vi "EnFlo_Turntable_Control.vi"(3 "Mode":T5, 5 "Traverse line In":T2={"Start X"=0.0, "Start Y"=nan, "Start Z"=nan, "End X"=nan, "End Y"=nan, "End Z"=nan, "nPoints"=0, "Spacing"=enum."N/A", "Filename"=path "  ---------", "Tunnel Speed"=nan, "Averaging time (mins)"=nan, "Extra Commands"="!Datum Image = Datum_Turntable.xls", "Carrier_1 Q (l/min)"=nan, "Carrier_2 Q (l/min)"=nan, "Trace Gas Concentration (%)"=nan, "Specific Arguments"="EnFlo_Turntable_Control.vi", "Comments"="", "Row No"=0, "Row Type Selector"=enum."Run VI Named:", "EstCompl"="09:40  12-04-2016", "Row Duration (mins)"=0.6666666666666666, "nValidPoints"=0, "Meas Setup File"="Trav_Cam_Picture.xls"} {"Carrier_2 Q (l/min)" format="%#.2f"; "Row Duration (mins)" format="%#.1f"; "Row No" min=0; "Trace Gas Concentration (%)" min=0.0 format="%#_4f"; "Carrier_1 Q (l/min)" format="%#.4f"; "Start X" format="%#.2f"; "Start Y" format="%#.2f"; "Start Z" format="%#.2f"; "End X" format="%#.2f"; "End Y" format="%#.2f"; "End Z" format="%#.2f"; "Tunnel Speed" format="%#.2f"; "Averaging time (mins)" min=0.0 format="%#.2f"}) -> (0 "Error Message":string, 1 "Status":T1, 2 "Traverse line Out":T2={"Start X"=0.0, "Start Y"=nan, "Start Z"=nan, "End X"=nan, "End Y"=nan, "End Z"=nan, "nPoints"=0, "Spacing"=enum."N/A", "Filename"=path "  ---------", "Tunnel Speed"=nan, "Averaging time (mins)"=nan, "Extra Commands"="!Datum Image = Datum_Turntable.xls", "Carrier_1 Q (l/min)"=nan, "Carrier_2 Q (l/min)"=nan, "Trace Gas Concentration (%)"=nan, "Specific Arguments"="EnFlo_Turntable_Control.vi", "Comments"="", "Row No"=0, "Row Type Selector"=enum."Run VI Named:", "EstCompl"="09:40  12-04-2016", "Row Duration (mins)"=0.6666666666666666, "nValidPoints"=0, "Meas Setup File"="Trav_Cam_Picture.xls"} {"Carrier_2 Q (l/min)" format="%#.2f"; "Row Duration (mins)" format="%#.1f"; "Row No" min=0; "Trace Gas Concentration (%)" min=0.0 format="%#_4f"; "Carrier_1 Q (l/min)" format="%#.4f"; "Start X" format="%#.2f"; "Start Y" format="%#.2f"; "Start Z" format="%#.2f"; "End X" format="%#.2f"; "End Y" format="%#.2f"; "End Z" format="%#.2f"; "Tunnel Speed" format="%#.2f"; "Averaging time (mins)" min=0.0 format="%#.2f"})   [LabVIEW 2022 SP3]
uses:
  Gen Trav/Traverse_cluster.ctl
  Gen Trav/Spacing.ctl
  Controls/Multi_run_mode.ctl
  Controls/User_Specific_mode.ctl
  Gen Trav/Multi_Run_Status.ctl
  Gen Trav/Trav_mode.ctl
  Controls/Tunnel_Coordinates.ctl
  ADAM Client/Sub VIs/ADAM Controls/Quick_local_ADAM_Table.ctl
  Controls/Setup.ctl
  Controls/Save_Data.ctl
  Camera Server/Camera enum/Camera resolution.ctl
  ADAM Client/Sub VIs/ADAM Controls/Update_scan_value.ctl
  Globals/Trav_pos_global.vi
  Globals/Extra_Commands_Global.vi
  Globals/Constants_global.vi
  Globals/Dynamic_call_global.ph.vi
panel:
  out "File Traverse Parking info comes from":path
  out "Traverse Parking Positions":string[][](table)
  out "Datum Filename":string
  out "Turntable image angle error":bool
  in  "max num of moves":i32=10
  out "Ratio of Error to move":sgl=0.8
  in  "stop":bool
  out "Turntable Angle":sgl format="%0.2f"
  out "Error in Turntable":sgl(graph)
  out "Angle Tolerance":sgl=0.02 format="%#_13g"
  out "Turntable Error":sgl
  out "Motor Position (Angle)":sgl(graph)
  out "Demanded Deg":sgl format="%#.4f"
  out "Correct Position":bool=TRUE
  out "Drive needs relaxing?":bool
  out "Relax Drive":sgl=0.25
  out "+ve Rotation":bool
  out "Motor Current Position":sgl
  # "X           Y          Z"
  # "Start"
  # "End"
  # "X           Y          Z"
  # "Start"
  # "End"
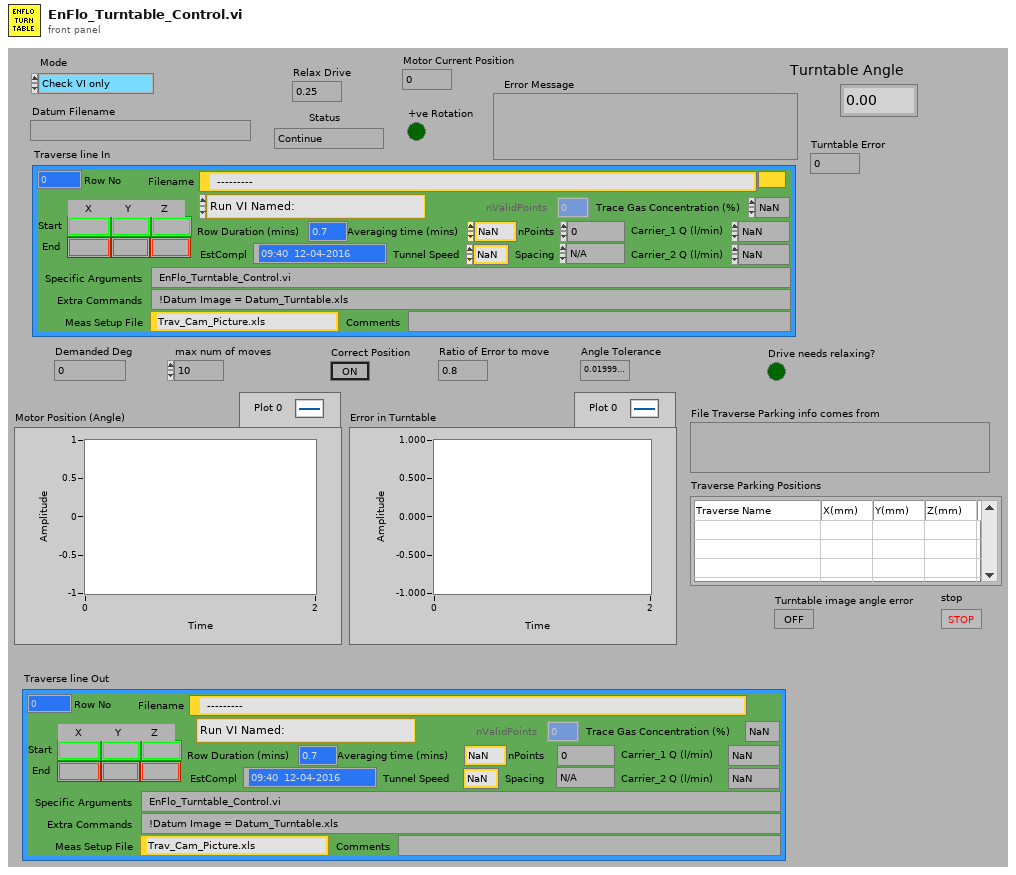
[diagram p1: front panel]
types:
  T1 = typedef "Multi_Run_Status.ctl" = enum16{"Continue", "Continue with Error", "Jump to Next Point", "Jump to Next Row", "Jump To Fall Back", "Terminate Run"}
  T2 = typedef "Traverse_cluster.ctl" = cluster{"Start X":sgl, "Start Y":sgl, "Start Z":sgl, "End X":sgl, "End Y":sgl, "End Z":sgl, "nPoints":i32, "Spacing":T3, "Filename":path, "Tunnel Speed":dbl, "Averaging time (mins)":dbl, "Extra Commands":string, "Carrier_1 Q (l/min)":dbl, "Carrier_2 Q (l/min)":dbl, "Trace Gas Concentration (%)":dbl, "Specific Arguments":string, "Comments":string, "Row No":i32, "Row Type Selector":T4, "EstCompl":string, "Row Duration (mins)":dbl, "nValidPoints":i32, "Meas Setup File":string}
  T3 = typedef "Spacing.ctl" = enum16{"Linear", "Log", "Gauss", "Specified", "N/A"}
  T4 = typedef "Multi_run_mode.ctl" = enum16{"Move Traverse Only", "Set Tunnel Speed Only", "Set Source Only", "Set Measurement Conditions", "Single Measurement", "Vertical Profile", "Lateral Profile", "Longitudinal Profile", "Multi-Axis Profile", "Explore Volume", "Auto Calibrate", "Meas Fast FID Bkgnd", "Check Beam Power", "Scanning Valve Measurement", "Run VI Named:", "Set ADAM Ch", "Wait (minutes)", "Send Message", "Synchronize With:", "Fall Back to this Row", "Turn Off Row Repeating", "Traverse 3D Volume", "Blank Row", "Jump to Fall Back Row"}
  T5 = typedef "User_Specific_mode.ctl" = enum16{"Check VI only", "Run VI"}
  T6 = typedef "Trav_mode.ctl" = enum16{"Move traverse", "Read traverse position", "Teach Position"}
  T7 = typedef "Tunnel_Coordinates.ctl" = enum16{"Work in Tunnel Coordinates", "Work in Model Coordinates"}
  T8 = typedef "Quick_local_ADAM_Table.ctl" = enum16{"Read Global", "Load Global From ADAM Table", "Write Global"}
  T9 = typedef "Save_Data.ctl" = enum16{"Save No Data", "Save Data"}
  T10 = typedef "Setup.ctl" = enum16{"Run Program", "Show Setup", "Save Current Setup", "Setup Front Panel"}
  T11 = typedef "Update_scan_value.ctl" = cluster{"Channel Name":string, "New Value":dbl, "!Auto_Off":bool}
  T12 = typedef "Camera resolution.ctl" = u8
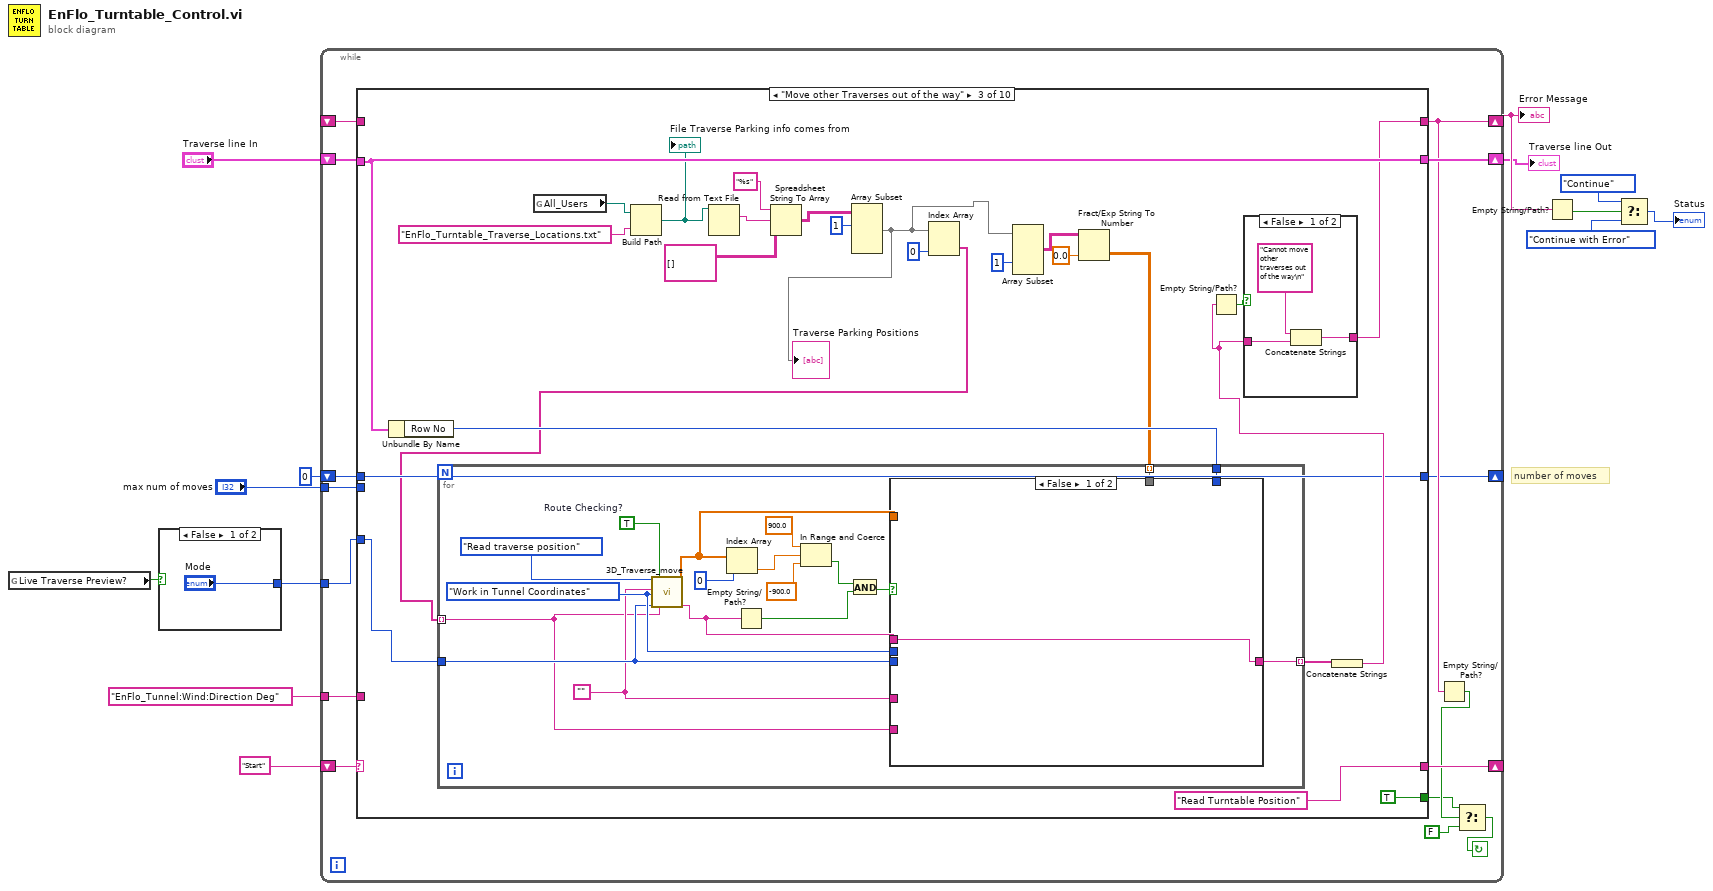
[diagram p0: block diagram]
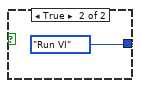
[diagram p2: hidden frame]
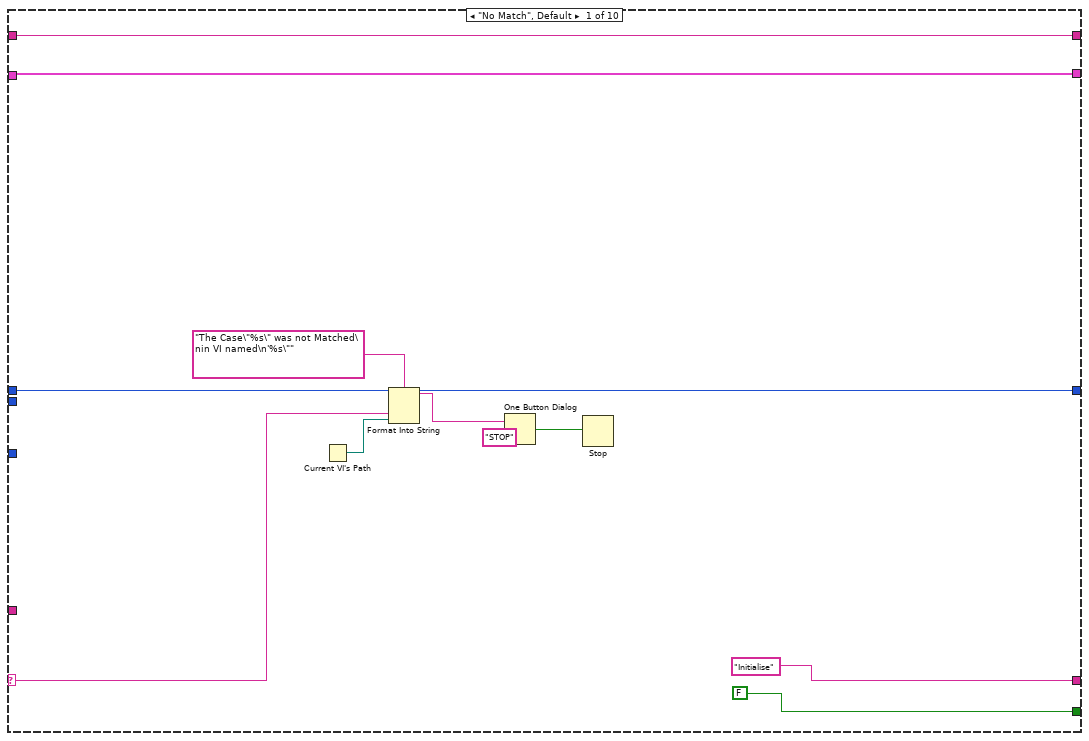
[diagram p3: hidden frame]
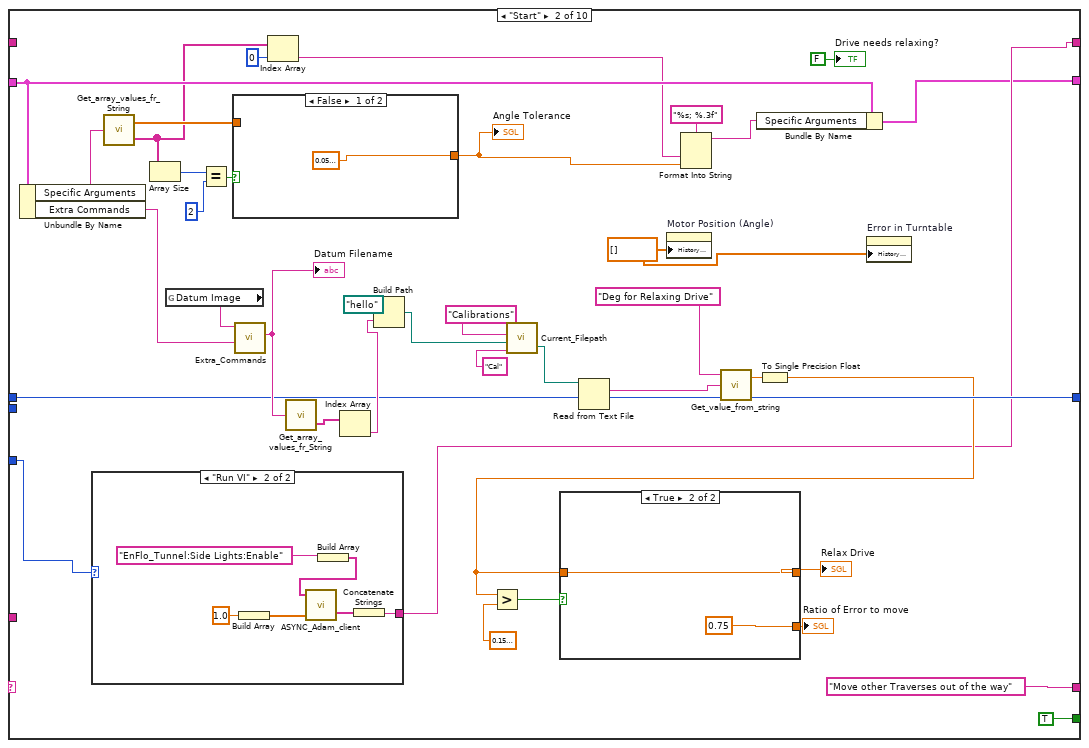
[diagram p4: hidden frame]
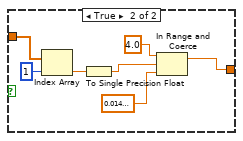
[diagram p5: hidden frame]
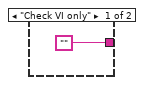
[diagram p6: hidden frame]
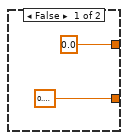
[diagram p7: hidden frame]
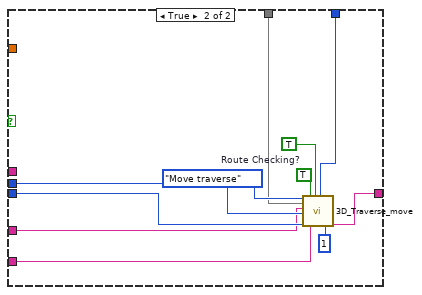
[diagram p9: hidden frame]
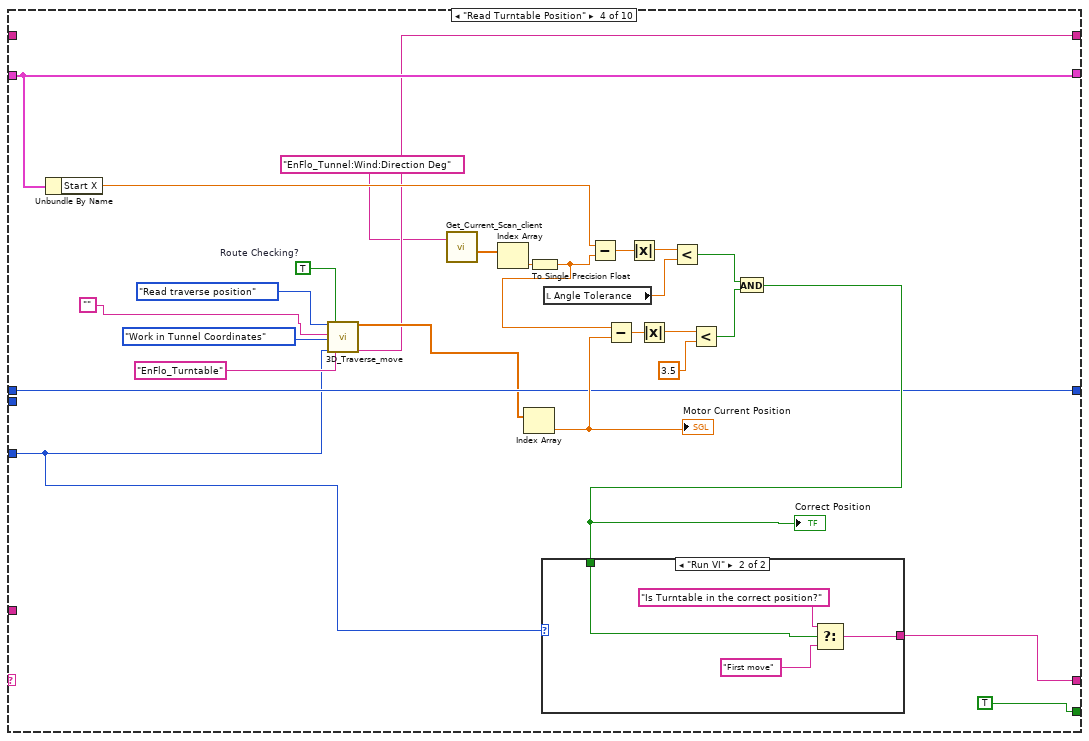
[diagram p10: hidden frame]
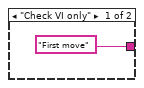
[diagram p11: hidden frame]
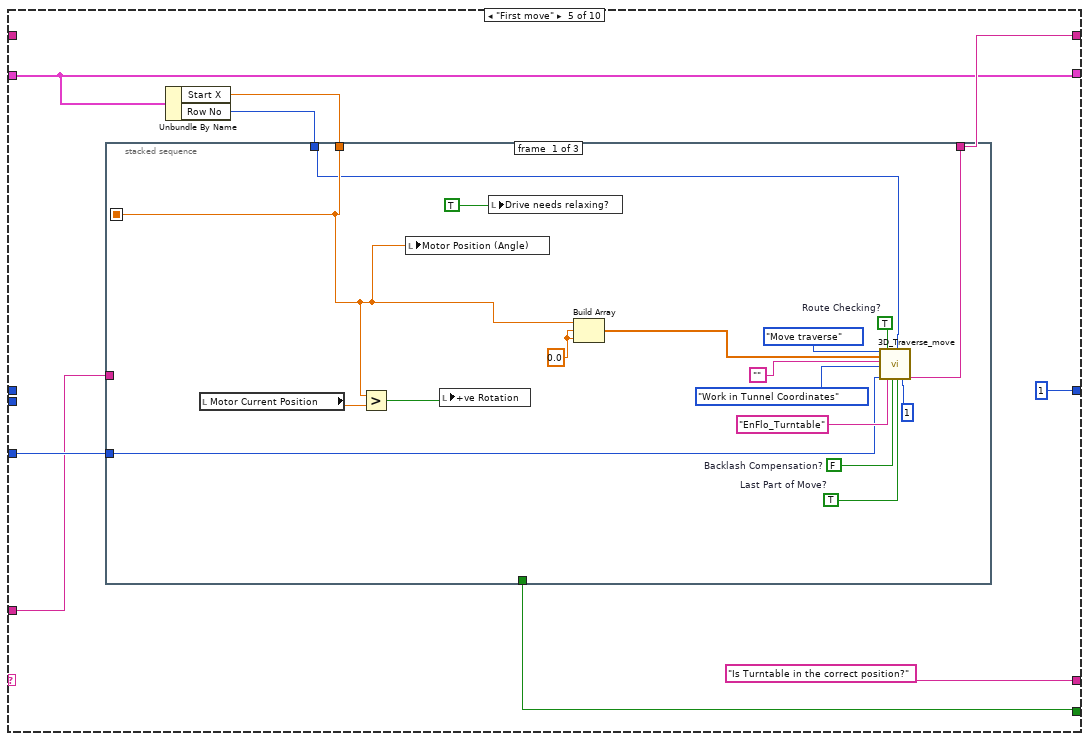
[diagram p12: hidden frame]
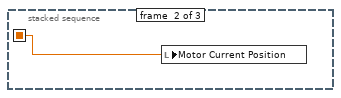
[diagram p13: hidden frame]
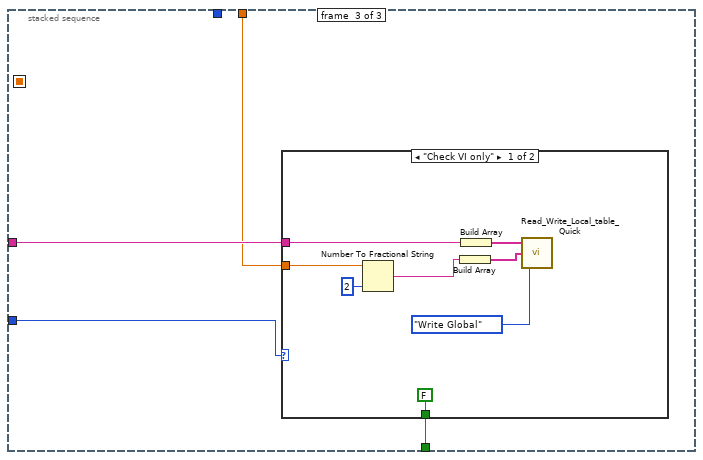
[diagram p14: hidden frame]
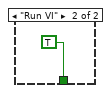
[diagram p15: hidden frame]
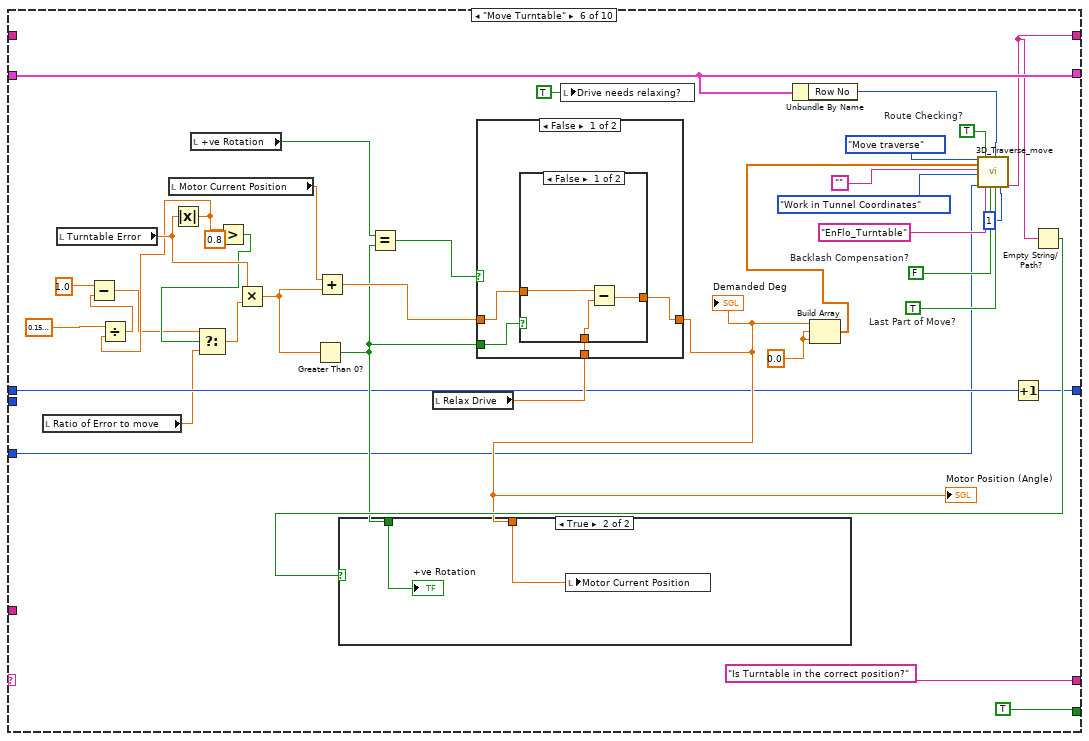
[diagram p16: hidden frame]
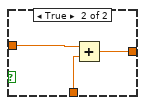
[diagram p17: hidden frame]
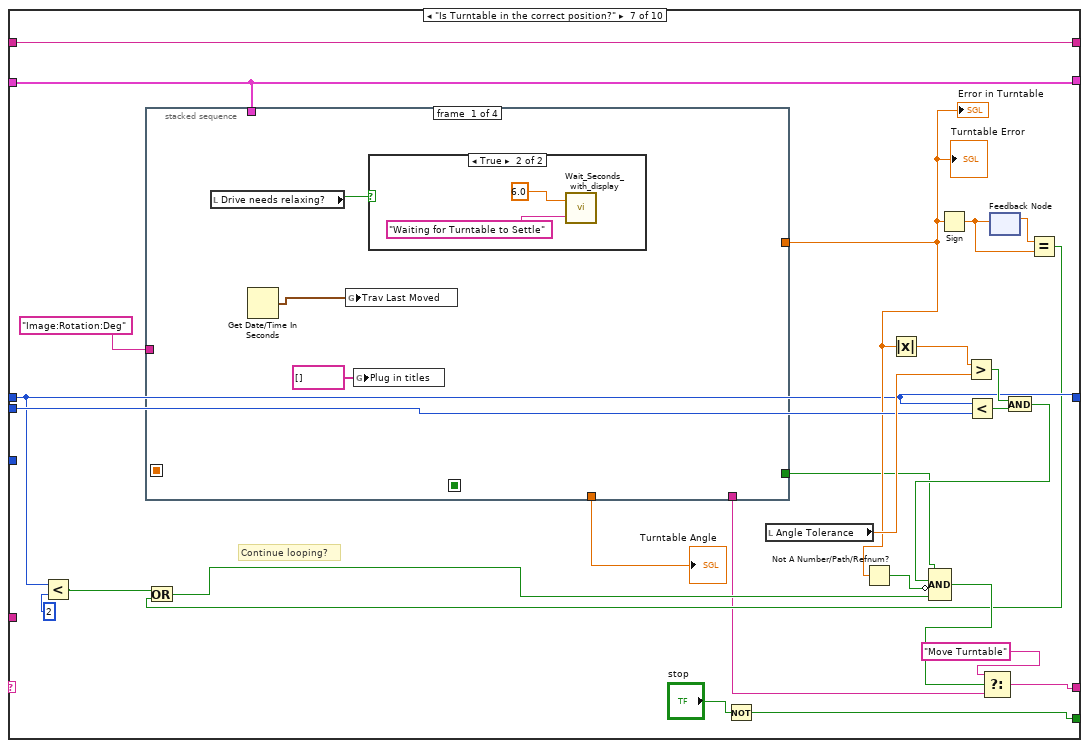
[diagram p20: hidden frame]
diagram:
  # "number of moves"
  n1 = global read "Trav_pos_global.vi" "Live Traverse Preview?"() -> (w4:bool)
  n2 = case shown="False" w4 {
    tunnel: ["Mode" User_Specific_mode."Run VI" ("Simulate/Run")] -> w3
    frame False {
    }
    frame True {
    }
  }
  n3 = while {
    shift-left: "Start" -> [w29]
    shift-right: [w30] -> _
    shift-right: [w27] -> w1
    shift-left: "Traverse line In" -> [w28]
    shift-right: [w25] -> w12
    shift-left: _ -> [w26]
    shift-right: [w20] -> _
    shift-left: 0 -> [w19]
    tunnel: "max num of moves" -> [w18]
    tunnel: w3 -> [w17]
    tunnel: "EnFlo_Tunnel:Wind:Direction Deg" -> [w16]
    stop <- w22 continue-if-true
    n4 = case shown="\"Move other Traverses out of the way\"" w29 {
      selector: w29 -> [w32 _ _ _ _ _ _ _ _ _]
      tunnel: [FALSE TRUE TRUE TRUE w192 TRUE w302 TRUE TRUE FALSE] -> w23
      tunnel: ["Initialise" "Move other Traverses out of the way" "Read Turntable Position" ("f") w182 "Is Turntable in the correct position?" "Is Turntable in the correct position?" w305 "Relax Turntable Drive" "Update Adam Table" "End"] -> w30
      tunnel: w17 -> [_ w57 w123 w159 w197 w230 _ w357 w383 _]
      tunnel: w28 -> [w34 w49 w118 w184 w195 w265 w301 w376 w399 w424]
      tunnel: [w34 w42 w118 w184 w195 w265 w301 w376 w399 w424] -> w27
      tunnel: [w33 w55 w115 w162 w196 w233 w288 w359 w386 w418] -> w25
      tunnel: w26 -> [w33 _ _ _ _ _ w288 _ _ w419]
      tunnel: [w31 w58 w114 w168 1 w253 w287 1 w397 w420] -> w20
      tunnel: w19 -> [w31 w58 w114 w168 _ w252 w287 _ w397 w420]
      tunnel: w18 -> [_ _ _ _ _ _ w299 _ _ _]
      tunnel: w16 -> [_ _ _ _ w190 _ _ _ _ w415]
      frame "No Match", Default {
        n5 = Current VI's Path() -> (path=w36:path)
        n6 = Format Into String(format string="The Case\"%s\" was not Matched\nin VI named\n'%s\"" ("Format String"), w32, w36) -> (resulting string=w39:string)  [unwired: 2 in, 1 out]
        n7 = One Button Dialog(message=w39, button name ("OK")="STOP") -> (true=w37:bool)
        n8 = Stop(stop? (T)=w37) -> ()
      }
      frame "Start" {
        w78 = dbl[] [] ("History Data")
        n9 = Unbundle By Name(w49) -> ("Specific Arguments"=w54:string, "Extra Commands"=w77:string)
        n10 = case shown="\"Run VI\"" w57 {
          tunnel: ["" w89] -> w55
          frame "Check VI only" {
          }
          frame "Run VI" {
            n11 = Build Array(1.0 ("element")) -> (w94:dbl[])
            n12 = Build Array("EnFlo_Tunnel:Side Lights:Enable") -> (w92:string[])
            n13 = call "ASYNC_Adam_client.vi"("Values"=w94, "Channel Names"=w92) -> ("Scan Comments"=w90:string[])  [unwired: 1 in, 1 out]
            n14 = Concatenate Strings(w90) -> (w89:string)
          }
        }
        n15 = call "Get_array_values_fr_String.vi"("String Value"=w54) -> ("Numeric Array"=w50:dbl[], "String array"=w48:string[])
        n16 = Array Size(array=w48) -> (size(s)=w53:i32)
        n17 = global read "Extra_Commands_Global.vi" "Datum Image"() -> (w69:string)
        n18 = Equal?(x=w53, y=2 ("x")) -> (x = y?=w51:bool)
        n19 = case shown="False" w51 {
          tunnel: [sgl 0.05 ("Angle Tolerance") w85] -> w45
          tunnel: w50 -> [_ w87]
          frame False {
          }
          frame True {
            n20 = Index Array(array=w87, index=1) -> (element=w82:dbl)
            n21 = To Single Precision Float(number=w82) -> (single precision float=w81:sgl)
            n22 = In Range and Coerce(upper limit=sgl 4.0, x=w81, lower limit=sgl 0.015) -> (coerced(x)=w85:sgl)  [unwired: 1 out]
          }
        }
        "Angle Tolerance" <- w45
        n23 = call "Extra_Commands.vi"("String to Search"=w77, "Command"=w69) -> ("String Value"=w65:string)  [unwired: 1 in, 4 out]
        "Datum Filename" <- w65
        n24 = Index Array(array=w48, index=0) -> (element=w46:string)
        n25 = call "Get_array_values_fr_String.vi"("String Value"=w65) -> ("String array"=w66:string[])  [unwired: 1 out]
        n26 = Index Array(array=w66) -> (element=w64:string)  [unwired: 1 in]
        n27 = Build Path(base path=path "hello", name or relative path=w64) -> (appended path=w70:path)
        n28 = call "Current_Filepath.vi"("Short_Name"="Cal" ("Data Type"), "Filename in"=w70, "Data Type"="Calibrations") -> ("Filename Out"=w74:path)  [unwired: 1 in, 1 out]
        n29 = Read from Text File(file (use dialog)=w74) -> (text=w67:string)  [unwired: 3 in, 3 out]
        n30 = property on="Motor Position (Angle)" class="WFChart (strict)"("History Data"=w78) -> ()  [unwired: 2 in, 2 out]
        n31 = Format Into String(format string="%s; %.3f", w46, w45) -> (resulting string=w43:string)  [unwired: 2 in, 1 out]
        n32 = call "Get_value_from_string.vi"("Input string"=w67, "Variable name"="Deg for Relaxing Drive" ("Label for characters")) -> ("Value"=w60:dbl)  [unwired: 1 in, 1 out]
        n33 = Bundle By Name(cluster=w49, "Specific Arguments"=w43) -> (w42:T2)
        n34 = To Single Precision Float(number=w60) -> (single precision float=w56:sgl)
        n35 = Greater?(x=w56, y=sgl 0.15) -> (0:w62:bool)
        n36 = case shown="True" w62 {
          tunnel: [sgl 0.0 ("Value") w98] -> w61
          tunnel: w56 -> [_ w98]
          tunnel: [sgl 0.6 ("Ratio of Error to move") sgl 0.75 ("Ratio of Error to move")] -> w59
          frame False {
          }
          frame True {
          }
        }
        "Relax Drive" <- w61
        "Ratio of Error to move" <- w59
        n37 = property on="Error in Turntable" class="WFChart (strict)"("History Data"=w78) -> ()  [unwired: 2 in, 2 out]
        "Drive needs relaxing?" <- FALSE ("Drive needs relaxing?")
      }
      frame "Move other Traverses out of the way" {
        n38 = Unbundle By Name(w118) -> ("Row No"=w122:i32)
        n39 = global read "Constants_global.vi" "All_Users"() -> (w113:path)
        n40 = Build Path(base path=w113, name or relative path="EnFlo_Turntable_Traverse_Locations.txt") -> (appended path=w111:path)
        "File Traverse Parking info comes from" <- w111
        n41 = Read from Text File(file (use dialog)=w111) -> (text=w110:string)  [unwired: 3 in, 3 out]
        n42 = Spreadsheet String To Array(format string="%s", spreadsheet string=w110, array type (2D Dbl)=string[][] []) -> (array=w108:string[][])  [unwired: 1 in]
        n43 = Array Subset(array=w108, index (row)=1 ("index")) -> (w99:string[][])  [unwired: 3 in]
        "Traverse Parking Positions" <- w99
        n44 = Index Array(array=w99, index (col)=0 ("disabled index (col)")) -> (element=w105:string[])  [unwired: 1 in]
        n45 = Array Subset(array=w99, index (col)=1 ("index")) -> (w102:string[][])  [unwired: 3 in]
        n46 = Fract/Exp String To Number(string=w102, default (0 dbl)=sgl 0.0 ("default (0 DBL)")) -> (number=w101:sgl[][])  [unwired: 2 in, 1 out]
        n47 = for {
          tunnel: w105 -> [w130] mode=indexing
          tunnel: w123 -> [w135]
          tunnel: w122 -> [w134]
          tunnel: [w133] -> w121 mode=indexing
          tunnel: w101 -> [w128] mode=indexing
          w129 = TRUE  # Route Checking?
          w131 = ""
          w136 = Tunnel_Coordinates."Work in Tunnel Coordinates" ("Work in Tunnel Coordinates")
          n48 = call "3D_Traverse_move.vi"("Mode"=Trav_mode."Read traverse position", "Extra command String"=w131, "Work in Tunnel Coordinates"=w136, "Simulate/Run"=w135, "Route Checking?"=w129, "Traverse name"=w130) -> ("Trav Position achieved"=w137:sgl[], "Error String"=w132:string)  [unwired: 10 in, 2 out]
          n49 = Index Array(array=w137, index=0) -> (element=w143:sgl)
          n50 = Empty String/Path?(string/path=w132) -> (empty?=w139:bool)
          n51 = In Range and Coerce(upper limit=sgl 900.0, x=w143, lower limit=sgl -900.0) -> (In Range?=w140:bool)  [unwired: 1 out]
          n52 = And(x=w140, y=w139) -> (x .and. y?=w138:bool)
          n53 = case shown="False" w138 {
            tunnel: w137 -> [_ _]
            tunnel: w136 -> [_ w156]
            tunnel: w135 -> [_ w155]
            tunnel: w130 -> [_ w148]
            tunnel: w134 -> [_ w153]
            tunnel: [w146 w150] -> w133
            tunnel: w132 -> [w146 _]
            tunnel: w131 -> [_ w149]
            tunnel: w128 -> [_ w147]
            frame False {
            }
            frame True {
              w154 = TRUE  # Route Checking?
              n54 = call "3D_Traverse_move.vi"("Mode"=Trav_mode."Move traverse", "Position"=w147, "Extra command String"=w149, "Work in Tunnel Coordinates"=w156, "Simulate/Run"=w155, "Route Checking?"=w154, "Traverse name"=w148, "Display Error"=TRUE ("Display Trav 2 Trav Error"), "Row Number"=w153, "Currently on Point"=1) -> ("Error String"=w150:string)  [unwired: 6 in, 3 out]
            }
          }
        }
        n55 = Concatenate Strings(w121) -> (w116:string)
        n56 = Empty String/Path?(string/path=w116) -> (empty?=w117:bool)
        n57 = case shown="False" w117 {
          tunnel: w116 -> [w125 w127]
          tunnel: [w124 w127] -> w115
          frame False {
            n58 = Concatenate Strings("Cannot move other traverses out of the way\n", w125) -> (w124:string)
          }
          frame True {
          }
        }
      }
      frame "Read Turntable Position" {
        w164 = TRUE  # Route Checking?
        n59 = Unbundle By Name(w184) -> ("Start X"=w183:sgl)
        n60 = call "3D_Traverse_move.vi"("Mode"=Trav_mode."Read traverse position", "Extra command String"="", "Work in Tunnel Coordinates"=Tunnel_Coordinates."Work in Tunnel Coordinates", "Simulate/Run"=w159, "Route Checking?"=w164, "Traverse name"="EnFlo_Turntable") -> ("Trav Position achieved"=w163:sgl[], "Error String"=w162:string)  [unwired: 10 in, 2 out]
        n61 = call "Get_Current_Scan_client.vi"("singleChannel"="EnFlo_Tunnel:Wind:Direction Deg") -> ("Numerical Values"=w181:dbl[])  [unwired: 1 in, 3 out]
        n62 = Index Array(array=w181) -> (element=w173:dbl)  [unwired: 1 in]
        n63 = Index Array(array=w163) -> (element=w170:sgl)  [unwired: 1 in]
        "Motor Current Position" <- w170
        n64 = To Single Precision Float(number=w173) -> (single precision float=w160:sgl)
        n65 = local read "Angle Tolerance"() -> (w174:sgl)
        n66 = Subtract(x=w183, y=w160) -> (x-y=w176:sgl)
        n67 = Subtract(x=w160, y=w170) -> (x-y=w180:sgl)
        n68 = Absolute Value(x=w176) -> (abs(x)=w175:sgl)
        n69 = Absolute Value(x=w180) -> (abs(x)=w179:sgl)
        n70 = Less?(x=w175, y=w174) -> (x < y?=w172:bool)
        n71 = Less?(x=w179, y=sgl 3.5) -> (x < y?=w177:bool)
        n72 = And(x=w172, y=w177) -> (x .and. y?=w171:bool)
        "Correct Position" <- w171
        n73 = case shown="\"Run VI\"" w159 {
          tunnel: ["First move" w189] -> w182
          tunnel: w171 -> [_ w186]
          frame "Check VI only" {
          }
          frame "Run VI" {
            n74 = Select(t="Is Turntable in the correct position?", s=w186, f="First move") -> (s? t:f=w189:string)
          }
        }
      }
      frame "First move" {
        n75 = Unbundle By Name(w195) -> ("Start X"=w194:sgl, "Row No"=w193:i32)
        n76 = stacked-sequence {
          seq-local: [w211 _ _] -> [_ w216 _]
          tunnel: w197 -> [w199 _ w220]
          tunnel: [w203 _ _] -> w196
          tunnel: w194 -> [w211 _ w217]
          tunnel: w193 -> [w200 _ _]
          tunnel: [_ _ w219] -> w192
          tunnel: w190 -> [_ _ w218]
          frame #0 {
            w207 = TRUE  # Route Checking?
            w205 = TRUE  # Last Part of Move?
            w215 = sgl 0.0 ("element")
            w206 = FALSE  # Backlash Compensation?
            n77 = local read "Motor Current Position"() -> (w214:sgl)
            n78 = Greater?(x=w211, y=w214) -> (0:w213:bool)
            n79 = local write "Motor Position (Angle)"(w211) -> ()
            n80 = local write "+ve Rotation"(w213) -> ()
            n81 = local write "Drive needs relaxing?"(TRUE ("Drive need relaxing?")) -> ()
            n82 = Build Array(w211, w215, w215) -> (w202:sgl[])
            n83 = call "3D_Traverse_move.vi"("Mode"=Trav_mode."Move traverse", "Position"=w202, "Extra command String"="", "Work in Tunnel Coordinates"=Tunnel_Coordinates."Work in Tunnel Coordinates", "Simulate/Run"=w199, "Route Checking?"=w207, "Traverse name"="EnFlo_Turntable", "Backlash Compensation?"=w206, "Row Number"=w200, "Last Part of Move?"=w205, "Currently on Point"=1) -> ("Error String"=w203:string)  [unwired: 5 in, 3 out]
          }
          frame #1 {
            n84 = local write "Motor Current Position"(w216) -> ()
          }
          frame #2 {
            n85 = case shown="\"Check VI only\"" w220 {
              tunnel: [FALSE TRUE] -> w219
              tunnel: w218 -> [w226 _]
              tunnel: w217 -> [w223 _]
              frame "Check VI only" {
                n86 = Number To Fractional String(number=w223, precision (6)=i16 2) -> (F-format string=w221:string)  [unwired: 2 in]
                n87 = Build Array(w221) -> (w224:string[])
                n88 = Build Array(w226) -> (w225:string[])
                n89 = call "Read_Write_Local_table_Quick.vi"("Mode"=Quick_local_ADAM_Table."Write Global", "String Values In"=w224, "Ch names In"=w225) -> ()  [unwired: 3 out]
              }
              frame "Run VI" {
              }
            }
          }
        }
      }
      frame "Move Turntable" {
        w238 = TRUE  # Route Checking?
        w236 = TRUE  # Last Part of Move?
        w237 = FALSE  # Backlash Compensation?
        w264 = sgl 0.0 ("element")
        n90 = local read "Ratio of Error to move"() -> (w248:sgl)
        n91 = local read "Turntable Error"() -> (w251:sgl)
        n92 = local read "Motor Current Position"() -> (w261:sgl)
        n93 = Absolute Value(x=w251) -> (abs(x)=w244:sgl)
        n94 = Divide(x=sgl 0.15, y=w244) -> (x/y=w243:sgl)
        n95 = Subtract(x=sgl 1.0, y=w243) -> (x-y=w242:sgl)
        n96 = local read "+ve Rotation"() -> (w258:bool)
        n97 = Greater?(x=w244, y=0.8) -> (0:w249:bool)
        n98 = Select(t=w242, s=w249, f=w248) -> (s? t:f=w247:sgl)
        n99 = Multiply(x=w251, y=w247) -> (x*y=w254:sgl)
        n100 = Greater Than 0?(x=w254) -> (x > 0?=w256:bool)
        n101 = Add(x=w261, y=w254) -> (x+y=w260:sgl)
        n102 = Equal?(x=w258, y=w256) -> (x = y?=w257:bool)
        n103 = local read "Relax Drive"() -> (w255:sgl)
        n104 = case shown="False" w257 {
          tunnel: w260 -> [w270 w278]
          tunnel: [w269 w278] -> w259
          tunnel: w256 -> [w271 _]
          tunnel: w255 -> [w268 _]
          frame False {
            n105 = case shown="False" w271 {
              tunnel: w270 -> [w274 w277]
              tunnel: [w272 w276] -> w269
              tunnel: w268 -> [w273 w275]
              frame False {
                n106 = Subtract(x=w274, y=w273) -> (x-y=w272:sgl)
              }
              frame True {
                n107 = Add(x=w277, y=w275) -> (x+y=w276:sgl)
              }
            }
          }
          frame True {
          }
        }
        "Demanded Deg" <- w259
        "Motor Position (Angle)" <- w259
        n108 = local write "Drive needs relaxing?"(TRUE ("Drive needs relaxing?")) -> ()
        n109 = Unbundle By Name(w265) -> ("Row No"=w232:i32)
        n110 = Build Array(w259, w264, w264) -> (w231:sgl[])
        n111 = call "3D_Traverse_move.vi"("Mode"=Trav_mode."Move traverse", "Position"=w231, "Extra command String"="", "Work in Tunnel Coordinates"=Tunnel_Coordinates."Work in Tunnel Coordinates", "Simulate/Run"=w230, "Route Checking?"=w238, "Traverse name"="EnFlo_Turntable", "Backlash Compensation?"=w237, "Row Number"=w232, "Last Part of Move?"=w236, "Currently on Point"=1) -> ("Error String"=w233:string)  [unwired: 5 in, 3 out]
        n112 = Increment(x=w252) -> (x+1=w253:i32)
        n113 = Empty String/Path?(string/path=w233) -> (empty?=w263:bool)
        n114 = case shown="True" w263 {
          tunnel: w256 -> [_ w280]
          tunnel: w259 -> [_ w279]
          frame False {
          }
          frame True {
            n115 = local write "Motor Current Position"(w279) -> ()
            "+ve Rotation" <- w280
          }
        }
      }
      frame "Is Turntable in the correct position?" {
        # "Continue looping?"
        n116 = Less?(x=w287, y=2) -> (x < y?=w285:bool)
        n117 = stacked-sequence {
          seq-local: [_ w323 _ _] -> [_ _ w335 _]
          seq-local: [_ _ w326 _] -> [_ _ _ w340]
          tunnel: w301 -> [_ w324 _ _]
          tunnel: [_ _ w333 _] -> w290
          tunnel: [_ _ w334 _] -> w292
          tunnel: "Image:Rotation:Deg" -> [_ _ w332 w341]
          tunnel: [_ _ _ w339] -> w282
          tunnel: [_ _ _ w338] -> w281
          frame #0 {
            n118 = local read "Drive needs relaxing?"() -> (w307:bool)
            n119 = Get Date/Time In Seconds() -> (seconds since 1Jan1904=w309:timestamp)
            n120 = global write "Trav_pos_global.vi" "Trav Last Moved"(w309) -> ()
            n121 = global write "Dynamic_call_global.ph.vi" "Plug in titles"(string[] [] ("Plug in titles")) -> ()
            n122 = case shown="True" w307 {
              frame False {
              }
              frame True {
                n123 = call "Wait_Seconds_with_display.vi"("Message"="Waiting for Turntable to Settle", "Seconds to wait"=6.0) -> ()  [unwired: 1 in, 1 out]
              }
            }
          }
          frame #1 {
            w313 = T12 0 items=["Low", "Med.", "High", "Max."] ("Camera Resolution")
            w322 = FALSE  # Remote control
            n124 = Unbundle By Name(w324) -> ("Comments"=w314:string, "Meas Setup File"=w317:string, "Start X"=w323:sgl)
            n125 = local read "Datum Filename"() -> (w312:string)
            n126 = Format Into String(format string="!Datum Image = %s;%.3f", w312, w323) -> (resulting string=w315:string)  [unwired: 2 in, 1 out]
            n127 = call "Code_to_run.vi"("Extra command String"=w315, "Current Row Comments"=w314, "Camera Resolution"=w313, "setup"=Setup."Run Program", "Remote control"=w322, "File"=Save_Data."Save Data", "Results Filename"=path "test/Meas_Turntable_Position.xls", "Averaging time (min)"=0.05, "Setup filename"=w317) -> ()  [unwired: 3 in, 4 out]
          }
          frame #2 {
            n128 = global read "Dynamic_call_global.ph.vi" "Plug in titles"() -> (w337:string[])
            n129 = global read "Dynamic_call_global.ph.vi" "Plug in values"() -> (w336:string[])
            n130 = Search 1D Array(1D array=w337, element=w332) -> (index of element=w329:i32)  [unwired: 1 in]
            n131 = Less Than 0?(x=w329) -> (x < 0?=w327:bool)
            n132 = Index Array(array=w336, index=w329) -> (element=w331:string)
            n133 = Equal?(x=w331, y="NaN") -> (x = y?=w328:bool)
            n134 = Or(x=w328, y=w327) -> (x .or. y?=w326:bool)
            "Turntable image angle error" <- w326
            n135 = Fract/Exp String To Number(string=w331, default (0 dbl)=sgl 0.0 ("default (0 DBL)")) -> (number=w334:sgl)  [unwired: 2 in, 1 out]
            n136 = Subtract(x=w335, y=w334) -> (x-y=w333:sgl)
          }
          frame #3 {
            n137 = case shown="True" w340 {
              tunnel: w341 -> [_ w349]
              tunnel: [w342 "No image feedback"] -> w338
              frame False {
                n138 = local read "Drive needs relaxing?"() -> (w345:bool)
                n139 = Select(t="Relax Turntable Drive", s=w345, f="Update Adam Table") -> (s? t:f=w342:string)
              }
              frame True {
                n140 = Format Into String(format string="Error in value of %s", w349) -> (resulting string=w348:string)  [unwired: 2 in, 1 out]
                n141 = Bundle By Name(cluster=errorcluster {"status"=FALSE, "code"=0, "source"=""} ("error in (no error)"), "status"=TRUE, "source"=w348) -> (w351:errorcluster)
                n142 = call "EnFlo_Error_Handler.vi"("error in (no error)"=w351, "Dialog Box (F)"=FALSE ("Dialog Box (T)")) -> ()  [unwired: 2 in, 2 out]
              }
            }
            n143 = Not(x=w340) -> (.not. x?=w339:bool)
          }
        }
        "Turntable Error" <- w290
        "Error in Turntable" <- w290
        "Turntable Angle" <- w292
        n144 = Not(x="stop") -> (.not. x?=w302:bool)
        n145 = local read "Angle Tolerance"() -> (w300:sgl)
        n146 = Not A Number/Path/Refnum?(number/path/refnum=w290) -> (NaN/Path/Refnum?=w289:bool)
        n147 = Absolute Value(x=w290) -> (abs(x)=w304:sgl)
        n148 = Sign(1:w290) -> (0:w294:sgl)
        n149 = Greater?(x=w304, y=w300) -> (0:w297:bool)
        n150 = Less?(x=w287, y=w299) -> (x < y?=w298:bool)
        n151 = feedback-in #1(w294) -> ()
        n152 = feedback #1() -> (w293:sgl)  [unwired: 1 in]
        n153 = And(x=w297, y=w298) -> (x .and. y?=w291:bool)
        n154 = Equal?(x=w293, y=w294) -> (x = y?=w284:bool)
        n155 = Or(x=w285, y=w284) -> (x .or. y?=w295:bool)
        n156 = Compound Arithmetic op=AND(w282, w291, invert w289, w295) -> (w296:bool)
        n157 = Select(t="Move Turntable", s=w296, f=w281) -> (s? t:f=w305:string)
      }
      frame "No image feedback" {
        w363 = TRUE  # Route Checking?
        w361 = TRUE  # Last Part of Move?
        w362 = FALSE  # Backlash Compensation?
        w371 = sgl 0.0 ("element")
        n158 = Unbundle By Name(w376) -> ("Start X"=w375:sgl, "Row No"=w354:i32)
        n159 = local read "+ve Rotation"() -> (w370:bool)
        n160 = local read "Relax Drive"() -> (w369:sgl)
        n161 = case shown="False" w370 {
          tunnel: w375 -> [w379 w381]
          tunnel: w369 -> [w378 w380]
          tunnel: [w377 w382] -> w368
          frame False {
            n162 = Subtract(x=w379, y=w378) -> (x-y=w377:sgl)
          }
          frame True {
            n163 = Add(x=w381, y=w380) -> (x+y=w382:sgl)
          }
        }
        n164 = Build Array(w368, w371, w371) -> (w355:sgl[])
        n165 = call "3D_Traverse_move.vi"("Mode"=Trav_mode."Move traverse", "Position"=w355, "Extra command String"="", "Work in Tunnel Coordinates"=Tunnel_Coordinates."Work in Tunnel Coordinates", "Simulate/Run"=w357, "Route Checking?"=w363, "Traverse name"="EnFlo_Turntable", "Backlash Compensation?"=w362, "Row Number"=w354, "Last Part of Move?"=w361, "Currently on Point"=1) -> ("Trav Position achieved"=w358:sgl[], "Error String"=w359:string)  [unwired: 5 in, 2 out]
        n166 = Index Array(array=w358) -> (element=w367:sgl)  [unwired: 1 in]
        n167 = local write "Motor Current Position"(w367) -> ()
      }
      frame "Relax Turntable Drive" {
        w392 = TRUE  # Route Checking?
        w390 = FALSE  # Last Part of Move?
        w391 = FALSE  # Backlash Compensation?
        w406 = sgl 0.0 ("element")
        n168 = local read "+ve Rotation"() -> (w405:bool)
        n169 = local read "Relax Drive"() -> (w398:sgl)
        n170 = case shown="False" w405 {
          tunnel: w398 -> [w408 w410]
          tunnel: [w408 w409] -> w403
          frame False {
          }
          frame True {
            n171 = Negate(x=w410) -> (-x=w409:sgl)
          }
        }
        n172 = local read "Motor Current Position"() -> (w401:sgl)
        n173 = Add(x=w401, y=w403) -> (x+y=w404:sgl)
        n174 = Build Array(w404, w406, w406) -> (w387:sgl[])
        n175 = Unbundle By Name(w399) -> ("Row No"=w384:i32)
        n176 = call "3D_Traverse_move.vi"("Mode"=Trav_mode."Move traverse", "Position"=w387, "Extra command String"="", "Work in Tunnel Coordinates"=Tunnel_Coordinates."Work in Tunnel Coordinates", "Simulate/Run"=w383, "Route Checking?"=w392, "Traverse name"="EnFlo_Turntable", "Backlash Compensation?"=w391, "Row Number"=w384, "Last Part of Move?"=w390, "Currently on Point"=1) -> ("Trav Position achieved"=w385:sgl[], "Error String"=w386:string)  [unwired: 5 in, 2 out]
        n177 = Index Array(array=w385) -> (element=w396:sgl)  [unwired: 1 in]
        n178 = local write "Drive needs relaxing?"(FALSE ("Drive needs relaxing?")) -> ()
        n179 = local write "Motor Current Position"(w396) -> ()
      }
      frame "Update Adam Table" {
        n180 = Unbundle By Name(w424) -> ("Start X"=w417:sgl)
        n181 = local read "Turntable image angle error"() -> (w412:bool)
        n182 = local read "Turntable Angle"() -> (w416:sgl)
        n183 = case shown="False" w412 {
          tunnel: w417 -> [w433 _]
          tunnel: w416 -> [w432 _]
          tunnel: [w431 w434] -> w411
          frame False {
            n184 = Not A Number/Path/Refnum?(number/path/refnum=w432) -> (NaN/Path/Refnum?=w430:bool)
            n185 = Select(t=w433, s=w430, f=w432) -> (s? t:f=w431:sgl)
          }
          frame True {
            n186 = local read "Motor Current Position"() -> (w434:sgl)
          }
        }
        n187 = Subtract(x=w416, y=w417) -> (x-y=w423:sgl)
        n188 = Absolute Value(x=w423) -> (abs(x)=w421:sgl)
        n189 = Greater?(x=w421, y=0.5) -> (0:w414:bool)
        n190 = Or(x=w412, y=w414) -> (x .or. y?=w413:bool)
        n191 = case shown="True" w413 {
          tunnel: w417 -> [_ w438]
          tunnel: w416 -> [_ w441]
          tunnel: w419 -> [w435 w440]
          tunnel: [w435 w439] -> w418
          tunnel: w412 -> [_ w437]
          tunnel: w411 -> [_ w436]
          frame False {
          }
          frame True {
            n192 = case shown="False" w437 {
              tunnel: w441 -> [w445 _]
              tunnel: w440 -> [w444 w449]
              tunnel: [w443 w448] -> w439
              tunnel: w438 -> [w442 _]
              tunnel: w436 -> [_ w447]
              frame False {
                n193 = Format Into String(format string="Desired Turntable angle is %.2f but achieived is %.2f.\n ", initial string=w444, w442, w445) -> (resulting string=w443:string)  [unwired: 1 in, 1 out]
              }
              frame True {
                n194 = Format Into String(format string="The Turntable angle had no image feedback, set to motor angle %.1f", initial string=w449, w447) -> (resulting string=w448:string)  [unwired: 1 in, 1 out]
              }
            }
          }
        }
        n195 = Bundle By Name(cluster=T11 {"Channel Name"="", "New Value"=0.0, "!Auto_Off"=FALSE} ("Update Scan Value Cluster"), "Channel Name"=w415, "New Value"=w411) -> (w427:T11)
        n196 = Build Array(w427) -> (w426:T11[])
        n197 = call "Update_Current_Value_client.vi"("Update array in"=w426) -> ()  [unwired: 1 in]
      }
    }
    n198 = Empty String/Path?(string/path=w25) -> (empty?=w24:bool)
    n199 = Select(t=w23, s=w24, f=FALSE) -> (s? t:f=w22:bool)
  }
  "Error Message" <- w12
  "Traverse line Out" <- w1
  n200 = Empty String/Path?(string/path=w12) -> (empty?=w11:bool)
  n201 = Select(t=Multi_Run_Status."Continue" ("Status"), s=w11, f=Multi_Run_Status."Continue with Error" ("Status")) -> (s? t:f=→"Status":T1)
